vi "Tree_ItemTag_Tests.vi"(11 "error in":errorcluster) -> (15 "error out":errorcluster)   [LabVIEW 2016, in "DronaTest.lvlib"]
uses:
  DronaTest.lvlib
  APIs/Stimulus/ControlValue/SetValueAuto.vi
  APIs/Stimulus/ControlValue/Controls/Tree/SetValueByItemTag.vi
  APIs/Assert/AssertControlValue/Equal.vi
  APIs/Get/GetControlRef/GetControlRefByPath.vi
  <vilib>/addons/_JKI Toolkits/Caraya/classes/Test/Test.lvclass
  Drona.lvlib
  <vilib>/SLL Toolkit/SLL Debug/SLL Debug.lvlib
  APIs/Assert/AssertControlValue/AssertControlValue.lvlib
  APIs/Stimulus/ControlValue/ControlValue.lvlib
  <vilib>/addons/_JKI Toolkits/Caraya/classes/Assert/Assert.lvclass
  APIs/Stimulus/ControlValue/Controls/Tree/StimulusTree.lvlib
  APIs/Get/GetControlRef/GetControlRef.lvlib
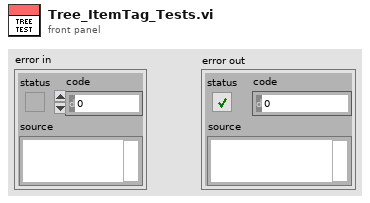
[diagram p1: front panel]
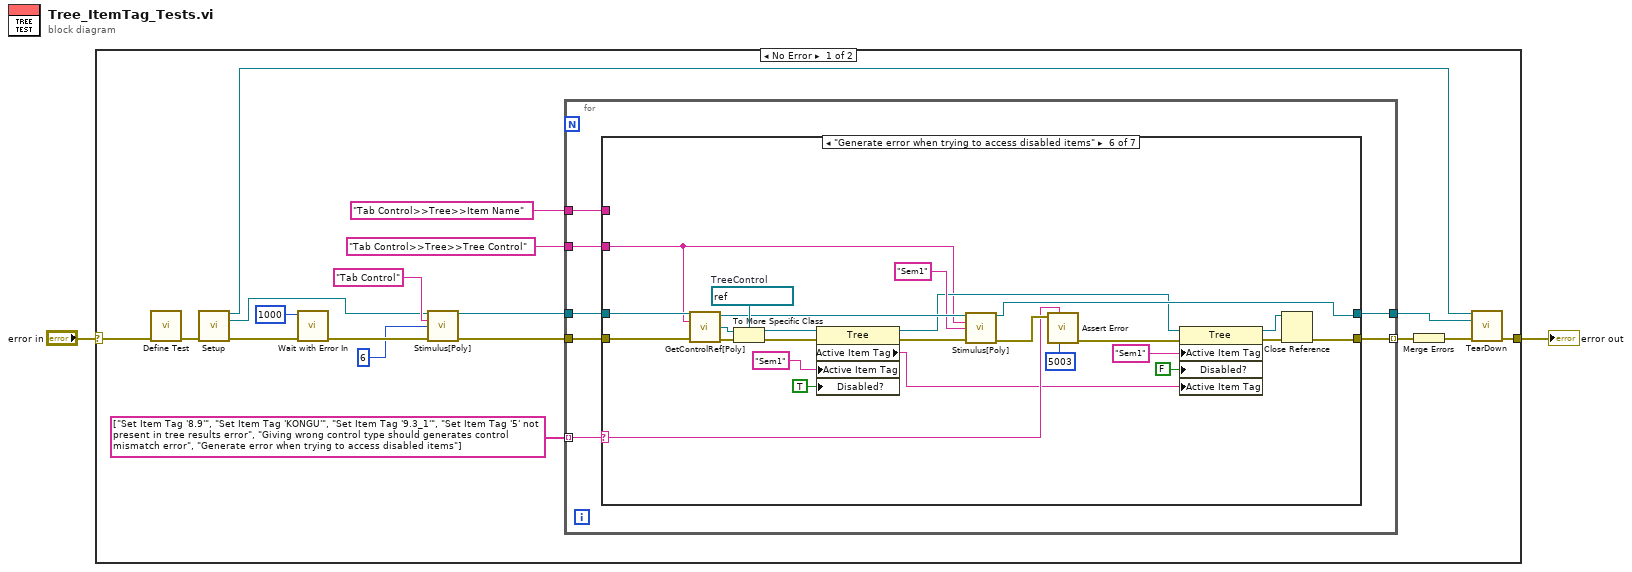
[diagram p0: block diagram]
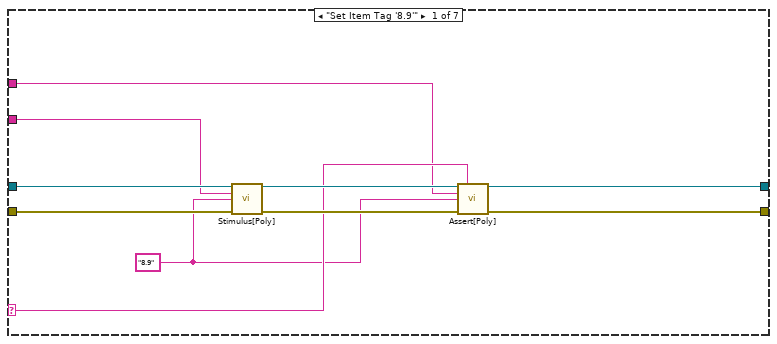
[diagram p2: hidden frame]
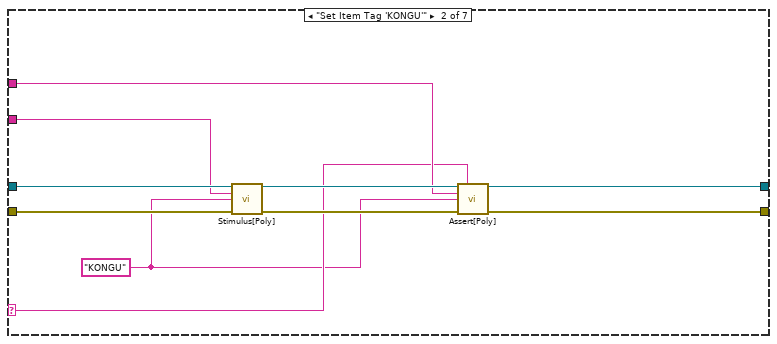
[diagram p3: hidden frame]
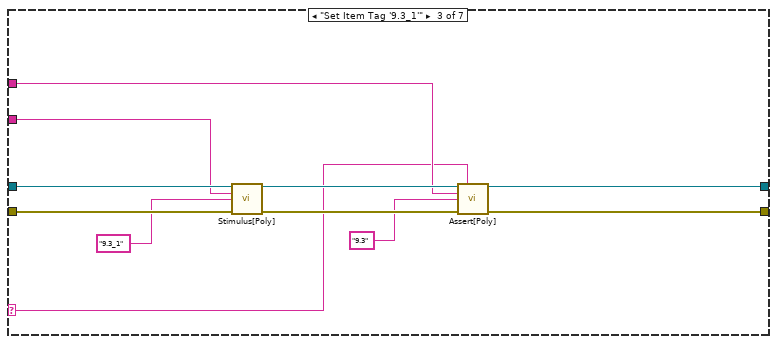
[diagram p4: hidden frame]
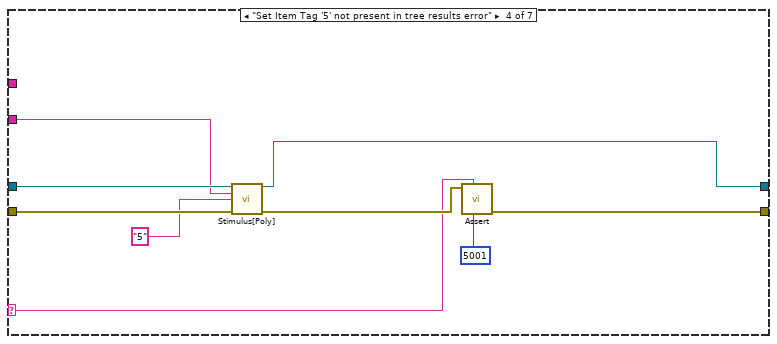
[diagram p5: hidden frame]
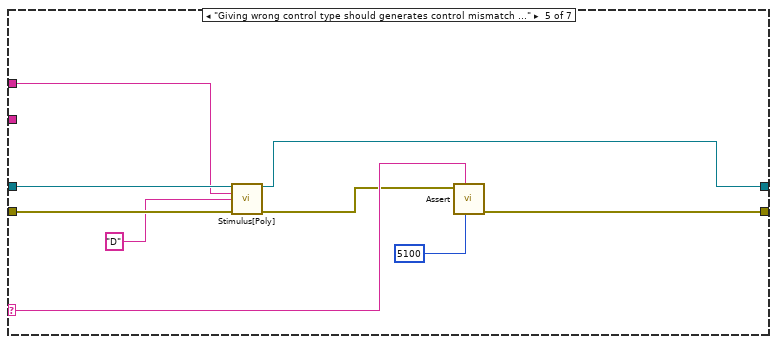
[diagram p6: hidden frame]
diagram:
  n1 = case shown="No Error" "error in" {
    selector: "error in" -> [w20 w104]
    tunnel: [w3 w104] -> w1
    frame No Error {
      n2 = call <vilib>:"Define Test.vi"("error in (no error)"=w20) -> ("error out"=w9:errorcluster)  [unwired: 9 in, 1 out]
      n3 = call "Setup.vi"("error in"=w9) -> ("Application Ref"=w4:refnum<vi>, "VI out"=w8:refnum<vi>, "error out"=w7:errorcluster)  [unwired: 12 in]
      n4 = call <vilib>:"Wait with Error In.vi"("error in (no error)"=w7, "milliseconds to wait"=u32 1000) -> ("error out"=w18:errorcluster)  [unwired: 9 in]
      n5 = call-poly "Stimulus[Poly].vi"("VI Reference In"=w8, "Control Path"="Tab Control", "Value (Signaling)"=6, "error in"=w18) -> ("VI Reference Out"=w14:refnum<vi>, "error out"=w17:errorcluster)  [unwired: 10 in]
      n6 = for {
        tunnel: w14 -> [w26]
        tunnel: "Tab Control>>Tree>>Tree Control" ("Control Path") -> [w25]
        tunnel: "Tab Control>>Tree>>Item Name" ("Control Path") -> [w24]
        tunnel: string[] ["Set Item Tag '8.9'", "Set Item Tag 'KONGU'", "Set Item Tag '9.3_1'", "Set Item Tag '5' not present in tree results error", "Giving wrong control type should generates control mismatch error", "Generate error when trying to access disabled items"] -> [w22] mode=indexing
        tunnel: [w21] -> w5
        tunnel: w17 -> [w27]
        tunnel: [w23] -> w10 mode=indexing
        n7 = case shown="\"Generate error when trying to access disabled items\"" w22 {
          selector: w22 -> [w31 w39 w50 w60 w73 w83 _]
          tunnel: w27 -> [w37 w47 w58 w67 w76 w101 w103]
          tunnel: w26 -> [w36 w46 w57 w66 w75 w99 w102]
          tunnel: w25 -> [w29 w43 w54 w65 _ w77 _]
          tunnel: w24 -> [w30 w42 w53 _ w68 _ _]
          tunnel: [w33 w41 w52 w64 w74 w91 w103] -> w23
          tunnel: [w32 w40 w51 w63 w72 w82 w102] -> w21
          frame "Set Item Tag '8.9'" {
            w28 = "8.9" ("Item Name")
            n8 = call-poly "Stimulus[Poly].vi"("VI Reference In"=w36, "Control Path"=w29, "Item Tag"=w28, "Error In"=w37) -> ("VI Reference Out"=w34:refnum<vi>, "Error Out"=w35:errorcluster)  [unwired: 10 in]
            n9 = call-poly "Assert[Poly].vi"("VI Reference In"=w34, "Test Label"=w31, "Control Path"=w30, "Control Value"=w28, "Error In"=w35) -> ("VI Reference Out"=w32:refnum<vi>, "Error Out"=w33:errorcluster)  [unwired: 8 in, 1 out]
          }
          frame "Set Item Tag 'KONGU'" {
            w38 = "KONGU" ("Item Name")
            n10 = call-poly "Stimulus[Poly].vi"("VI Reference In"=w46, "Control Path"=w43, "Item Tag"=w38, "Error In"=w47) -> ("VI Reference Out"=w44:refnum<vi>, "Error Out"=w45:errorcluster)  [unwired: 10 in]
            n11 = call-poly "Assert[Poly].vi"("VI Reference In"=w44, "Test Label"=w39, "Control Path"=w42, "Control Value"=w38, "Error In"=w45) -> ("VI Reference Out"=w40:refnum<vi>, "Error Out"=w41:errorcluster)  [unwired: 8 in, 1 out]
          }
          frame "Set Item Tag '9.3_1'" {
            n12 = call-poly "Stimulus[Poly].vi"("VI Reference In"=w57, "Control Path"=w54, "Item Tag"="9.3_1" ("Item Name"), "Error In"=w58) -> ("VI Reference Out"=w55:refnum<vi>, "Error Out"=w56:errorcluster)  [unwired: 10 in]
            n13 = call-poly "Assert[Poly].vi"("VI Reference In"=w55, "Test Label"=w50, "Control Path"=w53, "Control Value"="9.3" ("Item Name"), "Error In"=w56) -> ("VI Reference Out"=w51:refnum<vi>, "Error Out"=w52:errorcluster)  [unwired: 8 in, 1 out]
          }
          frame "Set Item Tag '5' not present in tree results error" {
            n14 = call-poly "Stimulus[Poly].vi"("VI Reference In"=w66, "Control Path"=w65, "Item Tag"="5" ("Item Name"), "Error In"=w67) -> ("VI Reference Out"=w63:refnum<vi>, "Error Out"=w61:errorcluster)  [unwired: 10 in]
            n15 = call-poly <vilib>:"Assert.vi"("error code (1)"=5001, "Label"=w60, "Error?"=w61) -> ("error out"=w64:errorcluster)  [unwired: 7 in, 1 out]
          }
          frame "Giving wrong control type should generates control mismatch error" {
            n16 = call-poly "Stimulus[Poly].vi"("VI Reference In"=w75, "Control Path"=w68, "Item Tag"="D" ("Item Name"), "Error In"=w76) -> ("VI Reference Out"=w72:refnum<vi>, "Error Out"=w70:errorcluster)  [unwired: 10 in]
            n17 = call-poly <vilib>:"Assert.vi"("error code (1)"=5100, "Label"=w73, "Error?"=w70) -> ("error out"=w74:errorcluster)  [unwired: 7 in, 1 out]
          }
          frame "Generate error when trying to access disabled items" {
            w96 = refnum<vi> refnum  # TreeControl
            n18 = call-poly "GetControlRef[Poly].vi"("VI Reference In"=w99, "Control Path"=w77, "error In"=w101) -> ("VI Reference Out"=w88:refnum<vi>, "Ctl Refnum"=w97:refnum<vi>, "error out"=w100:errorcluster)  [unwired: 10 in]
            n19 = To More Specific Class(target class=w96, reference=w97, error in=w100) -> (specific class reference=w95:refnum<vi>, error out=w98:errorcluster)
            n20 = property class="Tree"(reference=w95, error in=w98, "Active Item Tag"="Sem1" ("Active Item:Tag"), "Disabled?"=TRUE ("Active Item:Disabled?")) -> (reference out=w81:refnum<vi>, error out=w89:errorcluster, "Active Item Tag"=w80:string)
            n21 = call-poly "Stimulus[Poly].vi"("VI Reference In"=w88, "Control Path"=w77, "Item Tag"="Sem1", "Error In"=w89) -> ("VI Reference Out"=w82:refnum<vi>, "Error Out"=w86:errorcluster)  [unwired: 10 in]
            n22 = call <vilib>:"Assert Error.vi"("error code (1)"=5003, "Label"=w83, "Error?"=w86) -> ("error out"=w85:errorcluster)  [unwired: 7 in, 1 out]
            n23 = property class="Tree"(reference=w81, error in=w85, "Active Item Tag"="Sem1" ("Active Item:Tag"), "Disabled?"=FALSE ("Active Item:Disabled?"), "Active Item Tag"=w80) -> (reference out=w90:refnum<vi>, error out=w92:errorcluster)
            n24 = Close Reference(reference=w90, error in (no error)=w92) -> (error out=w91:errorcluster)
          }
          frame Default {
          }
        }
      }
      n25 = Merge Errors(w10) -> (w6:errorcluster)
      n26 = call "TearDown.vi"("Application Ref"=w4, "VI in"=w5, "error in (no error)"=w6) -> ("error out"=w3:errorcluster)  [unwired: 12 in]
    }
    frame Error {
    }
  }
  "error out" <- w1
